vi "Tilt.vi"(10 "liftDown?":bool) -> ()   [LabVIEW 2014]
uses:
  <vilib>/Rock Robotics/WPI/Solenoid/WPI_SolenoidValue.ctl
  Robot Global Data.vi
  <vilib>/Rock Robotics/WPI/Solenoid/WPI_SolenoidSetEnum.vi
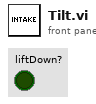
[diagram p1: front panel]
types:
  T1 = typedef "WPI_SolenoidValue.ctl" = enum16{"Off", "On", "Forward", "Reverse"}
  T2 = typedef "WPI_SolenoidDevRef.ctl" = cluster{"DevStatus":errorcluster, "Pneumatics Control Module":u8, "Forward Solenoid Channel":T3, "Reverse Solenoid Channel":T3}
  T3 = typedef "WPI_SolenoidChannel.ctl" = enum8{"Solenoid 0", "Solenoid 1", "Solenoid 2", "Solenoid 3", "Solenoid 4", "Solenoid 5", "Solenoid 6", "Solenoid 7", "Invalid"}
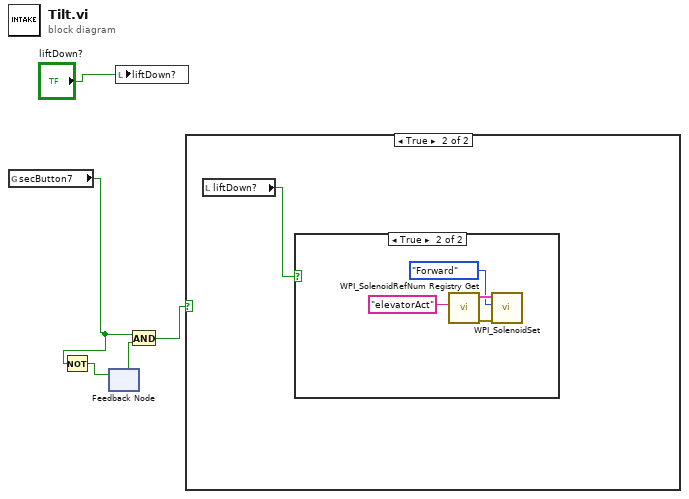
[diagram p0: block diagram]
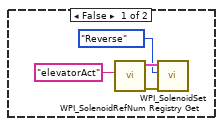
[diagram p3: hidden frame]
diagram:
  n1 = global read "Robot Global Data.vi" "secButton7"() -> (w5:bool)
  n2 = Not(x=w5) -> (.not. x?=w4:bool)
  n3 = feedback-in #1(w4) -> ()
  n4 = feedback #1() -> (w3:bool)  [unwired: 1 in]
  n5 = local write "liftDown?"("liftDown?") -> ()
  n6 = And(x=w5, y=w3) -> (x .and. y?=w1:bool)
  n7 = case shown="True" w1 {
    frame False {
    }
    frame True {
      n8 = local read "liftDown?"() -> (w6:bool)
      n9 = case shown="True" w6 {
        frame False {
          n10 = call <vilib>:"WPI_SolenoidRefNum Registry Get.vi"("refnum name"="elevatorAct") -> ("error out"=w8:errorcluster, "SolenoidDevRef"=w9:T2)  [unwired: 9 in]
          n11 = call-poly <vilib>:"WPI_SolenoidSet.vi"("error in (no error)"=w8, "Value"=WPI_SolenoidValue."Reverse", "SolenoidDevRef"=w9) -> ()  [unwired: 7 in, 2 out]
        }
        frame True {
          n12 = call <vilib>:"WPI_SolenoidRefNum Registry Get.vi"("refnum name"="elevatorAct") -> ("error out"=w12:errorcluster, "SolenoidDevRef"=w13:T2)  [unwired: 9 in]
          n13 = call-poly <vilib>:"WPI_SolenoidSet.vi"("error in (no error)"=w12, "Value"=WPI_SolenoidValue."Forward", "SolenoidDevRef"=w13) -> ()  [unwired: 7 in, 2 out]
        }
      }
    }
  }
